vi "Trigger Light Camera Sequence_MI.vi"(8 "error in (no error)":errorcluster, 10 "Trigger Light Camera Sequence":T1, 11 "Machine Interface Actor in":refnum<class "Machine Interface.lvclass">) -> (0 "error out":errorcluster, 3 "Machine Interface Actor out":refnum<class "Machine Interface.lvclass">)   [LabVIEW 2019, in "Machine Interface.lvclass"]
uses:
  Machine Interface.lvclass
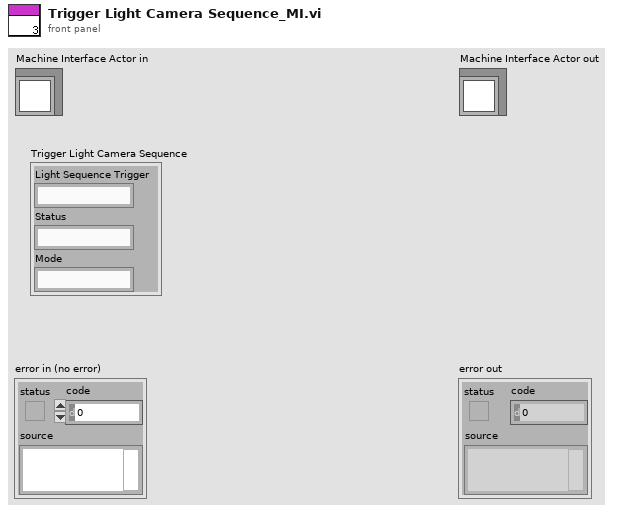
[diagram p1: front panel]
types:
  T1 = cluster{"Light Sequence Trigger":string, "Status":string, "Mode":string}
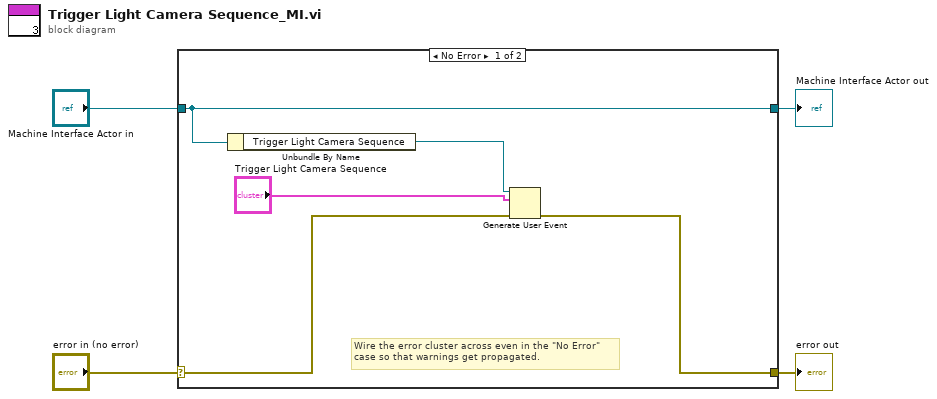
[diagram p0: block diagram]
diagram:
  n1 = case shown="No Error" "error in (no error)" {
    selector: "error in (no error)" -> [w6 w11]
    tunnel: [w5 w11] -> w3
    tunnel: [w8 w10] -> w1
    tunnel: "Machine Interface Actor in" -> [w8 w10]
    frame No Error {
      # "Wire the error cluster across even in the \"No Error\"\ncase so that warnings get propagated."
      n2 = Unbundle By Name(w8) -> ("Trigger Light Camera Sequence"=w7:refnum<user-event>)
      n3 = Generate User Event(user event=w7, event data cluster="Trigger Light Camera Sequence", error in=w6) -> (error out=w5:errorcluster)  [unwired: 1 in, 1 out]
    }
    frame Error {
    }
  }
  "error out" <- w3
  "Machine Interface Actor out" <- w1
